vi "Handle Timeout v2.vi"(8 "error in (no error)":errorcluster, 11 "cRIO Vacuum in":refnum<class "cRIO Vacuum.lvclass">) -> (0 "error out":errorcluster, 3 "cRIO Vacuum out":refnum<class "cRIO Vacuum.lvclass">)   [LabVIEW 2015, in "cRIO-Carbondioxide.lvlib" / "CO2-Actor.lvlib" / "cRIO Vacuum.lvclass"]
uses:
  cRIO Vacuum.lvclass
  cRIO Vacuum.lvclass/cRIO Vacuum.ctl
  Controls/Vacuum State Enumerator.ctl
  <vilib>/ptbypt/Time Domain.llb/Derivative x(t) PtByPt.vi
  <vilib>/ptbypt/NI_PtbyPt.lvlib
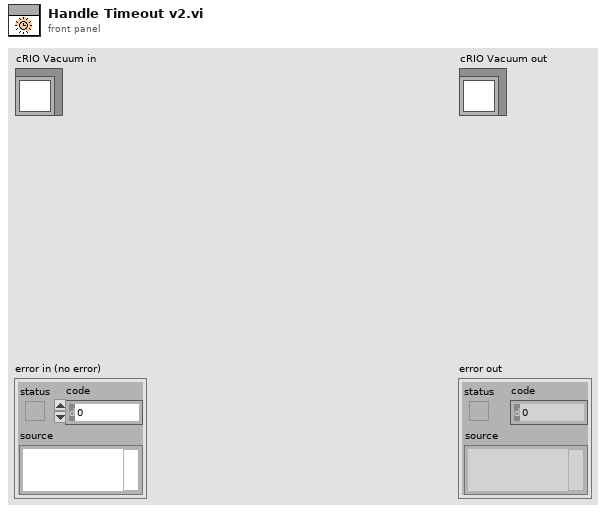
[diagram p1: front panel]
types:
  T1 = typedef "Vacuum State Enumerator.ctl" = enum16{"Pressure Rising", "Plateau", "Pressure Dropping", "Valley", "Low Valley", "Leak", "Unknown"}
  T2 = cluster{"Rizing":dbl, "Plateau":dbl, "Dropping":dbl, "Valley":dbl}
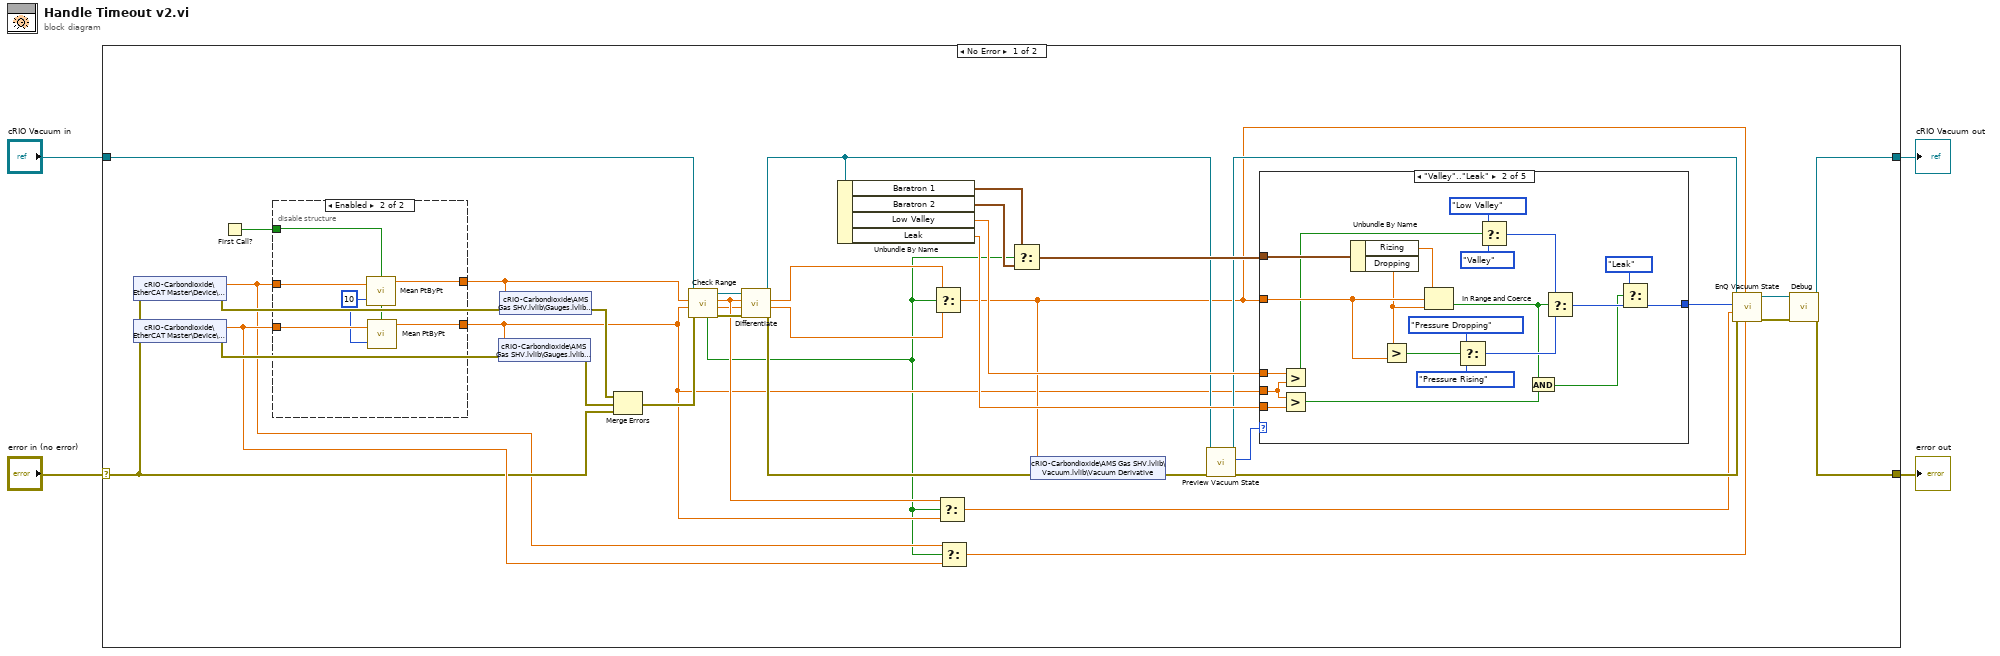
[diagram p0: block diagram]
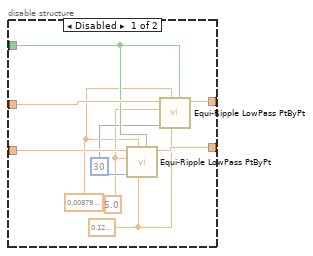
[diagram p2: hidden frame]
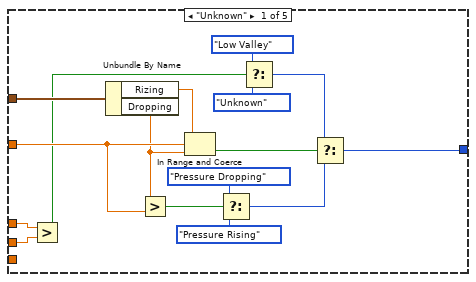
[diagram p3: hidden frame]
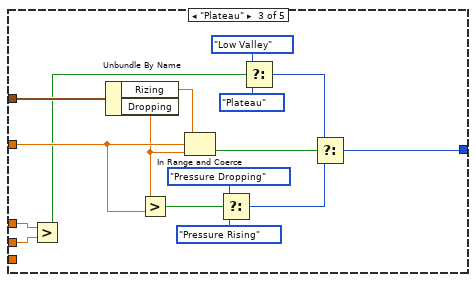
[diagram p4: hidden frame]
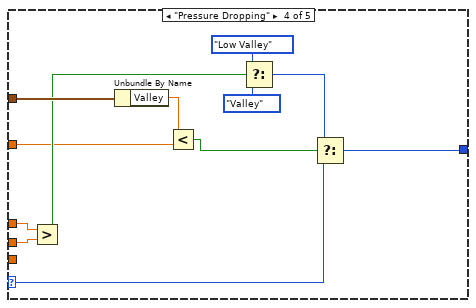
[diagram p5: hidden frame]
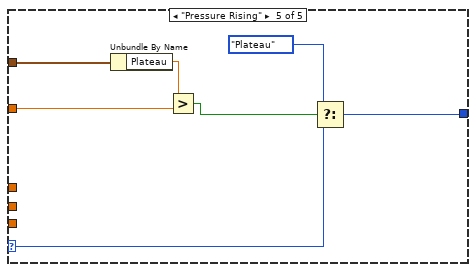
[diagram p6: hidden frame]
diagram:
  n1 = case shown="No Error" "error in (no error)" {
    selector: "error in (no error)" -> [w16 w131]
    tunnel: [w39 w131] -> w3
    tunnel: [w40 w130] -> w1
    tunnel: "cRIO Vacuum in" -> [w13 w130]
    frame No Error {
      n2 = shared-variable "cRIO-Carbondioxide\\EtherCAT Master\\Device\\Mod7\\Baratron 1"(error in=w16) -> (w15:dbl, error out=w41:errorcluster)
      n3 = shared-variable "cRIO-Carbondioxide\\EtherCAT Master\\Device\\Mod7\\Baratron 2"(error in=w16) -> (w38:dbl, error out=w42:errorcluster)
      n4 = First Call?() -> (First Call?: T/F=w14:bool)
      n5 = disable-structure shown="Enabled" {
        disable-tunnel: w38 -> [w51 w55]
        disable-tunnel: [w50 w54] -> w7
        disable-tunnel: w15 -> [w49 w57]
        disable-tunnel: [w48 w56] -> w9
        disable-tunnel: w14 -> [w47 w53]
        frame Disabled {
          w46 = 30 ("# of taps")
          w44 = 0.00879999999999983 ("pass freq")
          w43 = 0.1299999999999999 ("stop freq")
          w45 = 5.0 ("sampling freq: fs")
          n6 = call <vilib>:"Equi-Ripple LowPass PtByPt.vi"("initialize"=w47, "stop freq"=w43, "pass freq"=w44, "# of taps"=w46, "sampling freq: fs"=w45, "x"=w51) -> ("Filtered x"=w50:dbl)  [unwired: 3 in, 1 out]
          n7 = call <vilib>:"Equi-Ripple LowPass PtByPt.vi"("initialize"=w47, "stop freq"=w43, "pass freq"=w44, "# of taps"=w46, "sampling freq: fs"=w45, "x"=w49) -> ("Filtered x"=w48:dbl)  [unwired: 3 in, 1 out]
        }
        frame Enabled {
          w52 = 10 ("sample length")
          n8 = call <vilib>:"Mean PtByPt.vi"("x"=w57, "sample length"=w52, "initialize"=w53) -> ("mean"=w56:dbl)  [unwired: 1 in, 1 out]
          n9 = call <vilib>:"Mean PtByPt.vi"("x"=w55, "sample length"=w52, "initialize"=w53) -> ("mean"=w54:dbl)  [unwired: 1 in, 1 out]
        }
      }
      n10 = shared-variable "cRIO-Carbondioxide\\AMS Gas SHV.lvlib\\Gauges.lvlib\\Baratron 2"(w7, error in=w42) -> (error out=w37:errorcluster)
      n11 = shared-variable "cRIO-Carbondioxide\\AMS Gas SHV.lvlib\\Gauges.lvlib\\Baratron 1"(w9, error in=w41) -> (error out=w22:errorcluster)
      n12 = Merge Errors(w22, w37, w16) -> (w11:errorcluster)
      n13 = call "Check Range.vi"("error in (no error)"=w11, "Baratron 2"=w7, "Baratron 1"=w9, "cRIO Vacuum in"=w13) -> ("error out"=w10:errorcluster, "Baratron 2"=w6:dbl, "Baratron 1"=w8:dbl, "cRIO Vacuum out"=w12:refnum<class "cRIO Vacuum.lvclass">, "B2 out of range"=w5:bool)  [unwired: 3 in]
      n14 = call "Differentiate.vi"("error in (no error)"=w10, "Baratron 2"=w6, "Baratron 1"=w8, "cRIO Vacuum in"=w12) -> ("error out"=w19:errorcluster, "d/dt 2"=w35:dbl, "d/dt 1"=w36:dbl, "cRIO Vacuum out"=w23:refnum<class "cRIO Vacuum.lvclass">)  [unwired: 4 in]
      n15 = Unbundle By Name(w23) -> ("Baratron 1"=w34:T2, "Baratron 2"=w33:T2, "Low Valley"=w30:dbl, "Leak"=w29:dbl)
      n16 = Select(t=w36, s=w5, f=w35) -> (s? t:f=w17:dbl)
      n17 = Select(t=w8, s=w5, f=w7) -> (s? t:f=w25:dbl)
      n18 = Select(t=w15, s=w5, f=w38) -> (s? t:f=w24:dbl)
      n19 = Select(t=w34, s=w5, f=w33) -> (s? t:f=w32:T2)
      n20 = shared-variable "cRIO-Carbondioxide\\AMS Gas SHV.lvlib\\Vacuum.lvlib\\Vacuum Derivative"(w17, error in=w19) -> (error out=w18:errorcluster)
      n21 = call "Preview Vacuum State.vi"("error in (no error)"=w18, "cRIO Vacuum in"=w23) -> ("error out"=w28:errorcluster, "Vacuum State"=w31:T1, "cRIO Vacuum out"=w26:refnum<class "cRIO Vacuum.lvclass">)  [unwired: 3 in, 4 out]
      n22 = case shown="\"Valley\"..\"Leak\"" w31 {
        selector: w31 -> [_ _ _ w111 w124]
        tunnel: w32 -> [w73 w94 w110 w122 w129]
        tunnel: w17 -> [w69 w91 w106 w113 w126]
        tunnel: w7 -> [w63 w82 w100 w120 _]
        tunnel: w30 -> [w64 w86 w101 w121 _]
        tunnel: [w58 w77 w95 w115 w128] -> w27
        tunnel: w29 -> [_ w81 _ _ _]
        frame "Unknown" {
          n23 = Greater?(x=w64, y=w63) -> (0:w62:bool)
          n24 = Unbundle By Name(w73) -> ("Rizing"=w72:dbl, "Dropping"=w68:dbl)
          n25 = Greater?(x=w68, y=w69) -> (0:w70:bool)
          n26 = In Range and Coerce(upper limit=w72, x=w69, lower limit=w68) -> (In Range?=w71:bool)  [unwired: 1 out]
          n27 = Select(t=Vacuum_State_Enumerator."Pressure Dropping" ("Vacuum State"), s=w70, f=Vacuum_State_Enumerator."Pressure Rising") -> (s? t:f=w67:T1)
          n28 = Select(t=Vacuum_State_Enumerator."Low Valley", s=w62, f=Vacuum_State_Enumerator."Unknown" ("Vacuum State")) -> (s? t:f=w59:T1)
          n29 = Select(t=w59, s=w71, f=w67) -> (s? t:f=w58:T1)
        }
        frame "Valley".."Leak" {
          n30 = Greater?(x=w86, y=w82) -> (0:w85:bool)
          n31 = Greater?(x=w82, y=w81) -> (0:w76:bool)
          n32 = Unbundle By Name(w94) -> ("Rizing"=w93:dbl, "Dropping"=w90:dbl)
          n33 = Greater?(x=w90, y=w91) -> (0:w92:bool)
          n34 = In Range and Coerce(upper limit=w93, x=w91, lower limit=w90) -> (In Range?=w75:bool)  [unwired: 1 out]
          n35 = Select(t=Vacuum_State_Enumerator."Pressure Dropping" ("Vacuum State"), s=w92, f=Vacuum_State_Enumerator."Pressure Rising") -> (s? t:f=w89:T1)
          n36 = Select(t=Vacuum_State_Enumerator."Low Valley", s=w85, f=Vacuum_State_Enumerator."Valley" ("Vacuum State")) -> (s? t:f=w79:T1)
          n37 = And(x=w75, y=w76) -> (x .and. y?=w74:bool)
          n38 = Select(t=w79, s=w75, f=w89) -> (s? t:f=w78:T1)
          n39 = Select(t=Vacuum_State_Enumerator."Leak", s=w74, f=w78) -> (s? t:f=w77:T1)
        }
        frame "Plateau" {
          n40 = Greater?(x=w101, y=w100) -> (0:w99:bool)
          n41 = Unbundle By Name(w110) -> ("Rizing"=w109:dbl, "Dropping"=w105:dbl)
          n42 = Greater?(x=w105, y=w106) -> (0:w107:bool)
          n43 = In Range and Coerce(upper limit=w109, x=w106, lower limit=w105) -> (In Range?=w108:bool)  [unwired: 1 out]
          n44 = Select(t=Vacuum_State_Enumerator."Pressure Dropping" ("Vacuum State"), s=w107, f=Vacuum_State_Enumerator."Pressure Rising") -> (s? t:f=w104:T1)
          n45 = Select(t=Vacuum_State_Enumerator."Low Valley", s=w99, f=Vacuum_State_Enumerator."Plateau" ("Vacuum State")) -> (s? t:f=w96:T1)
          n46 = Select(t=w96, s=w108, f=w104) -> (s? t:f=w95:T1)
        }
        frame "Pressure Dropping" {
          n47 = Greater?(x=w121, y=w120) -> (0:w119:bool)
          n48 = Unbundle By Name(w122) -> ("Valley"=w114:dbl)
          n49 = Less?(x=w114, y=w113) -> (x < y?=w112:bool)
          n50 = Select(t=Vacuum_State_Enumerator."Low Valley", s=w119, f=Vacuum_State_Enumerator."Valley" ("Vacuum State")) -> (s? t:f=w116:T1)
          n51 = Select(t=w116, s=w112, f=w111) -> (s? t:f=w115:T1)
        }
        frame "Pressure Rising" {
          n52 = Unbundle By Name(w129) -> ("Plateau"=w127:dbl)
          n53 = Greater?(x=w127, y=w126) -> (0:w125:bool)
          n54 = Select(t=Vacuum_State_Enumerator."Plateau", s=w125, f=w124) -> (s? t:f=w128:T1)
        }
      }
      n55 = call "EnQ Vacuum State.vi"("Raw Pressure"=w24, "d/dt"=w17, "error in (no error)"=w28, "Pressure"=w25, "State"=w27, "cRIO Vacuum in"=w26) -> ("error out"=w20:errorcluster, "cRIO Vacuum out"=w21:refnum<class "cRIO Vacuum.lvclass">)  [unwired: 4 out]
      n56 = call "Debug.vi"("error in (no error)"=w20, "cRIO Vacuum in"=w21) -> ("error out"=w39:errorcluster, "cRIO Vacuum out"=w40:refnum<class "cRIO Vacuum.lvclass">)  [unwired: 8 in]
    }
    frame Error {
    }
  }
  "error out" <- w3
  "cRIO Vacuum out" <- w1
